vi "Enable Custom Device.vi"(8 "error in":errorcluster, 11 "Ballard MIL-STD 1553 custom device in":T1 format="%.0x") -> (0 "error out":errorcluster, 3 "Ballard MIL-STD 1553 custom device out":T1 format="%.0x")   [LabVIEW 2023, in "Ballard MIL-STD-1553 Scripting.lvlib"]
uses:
  Ballard MIL-STD-1553 Scripting.lvlib
  <vilib>/NI VeriStand/Custom Device API/Custom Device API.lvlib
  Constants.vi
  NationalInstruments.VeriStand.SystemDefinitionAPI
  <vilib>/NI VeriStand/Custom Device API/Custom Device Item Ref.ctl
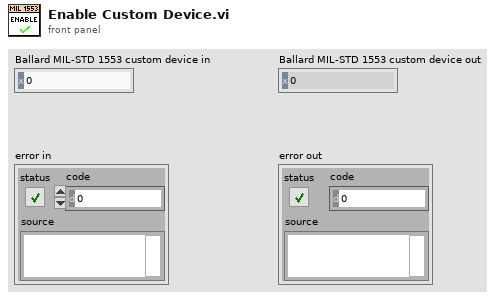
[diagram p1: front panel]
types:
  T1 = typedef "Custom Device API.lvlib/Custom Device Item Ref.ctl" = u64
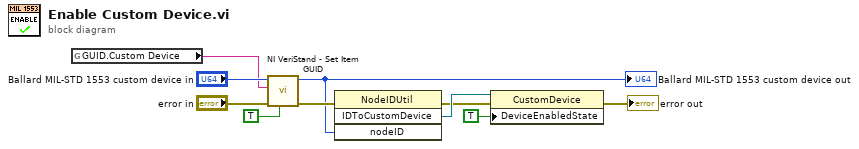
[diagram p0: block diagram]
diagram:
  n1 = global read "Constants.vi" "GUID.Custom Device"() -> (w9:string)
  n2 = call <vilib>:"NI VeriStand - Set Item GUID.vi"("Refresh System Explorer Tree? (F)"=TRUE, "error in (no error)"="error in", "GUID"=w9, "Item Ref in"="Ballard MIL-STD 1553 custom device in") -> ("error out"=w6:errorcluster, "Item Ref out"=w5:T1)  [unwired: 6 in]
  "Ballard MIL-STD 1553 custom device out" <- w5
  n3 = invoke class="NodeIDUtil" method="IDToCustomDevice"(error in=w6, "nodeID"=w5) -> (error out=w3:errorcluster, "IDToCustomDevice"=w4:refnum<k24>)  [unwired: 2 in, 2 out]
  n4 = property class="CustomDevice"(reference=w4, error in=w3, "DeviceEnabledState"=TRUE) -> (error out=→"error out":errorcluster)  [unwired: 1 out]
